vi "RTM Frames to be Faulted.vi"(8 "error in (no error)":errorcluster) -> (0 "error out":errorcluster)   [LabVIEW 2018, in "CAN Gateway System Explorer.lvlib"]
uses:
  CAN Gateway System Explorer.lvlib
  <vilib>/NI Veristand/Custom Device API/Custom Device Item Ref.ctl
  <vilib>/NI Veristand/Custom Device API/Custom Device API.lvlib
panel:
  out "Node Ptr 2":T1 format="%.0x"
  in  "Node Ptr":T1 format="%.0x"
  in  "Tag":string
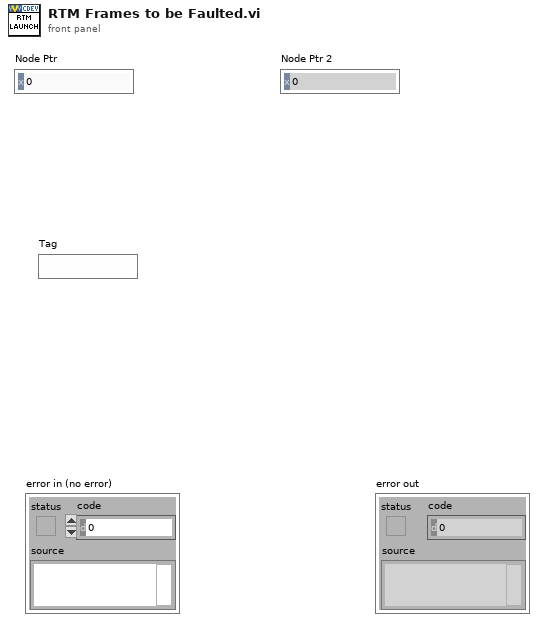
[diagram p1: front panel]
types:
  T1 = typedef "Custom Device API.lvlib/Custom Device Item Ref.ctl" = u64
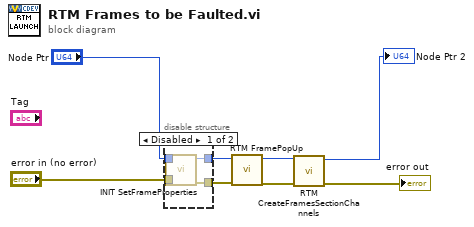
[diagram p0: block diagram]
diagram:
  n1 = disable-structure shown="Disabled" {
    disable-tunnel: [w12 w13] -> w5
    disable-tunnel: "error in (no error)" -> [w11 w13]
    disable-tunnel: "Node Ptr" -> [w10 w14]
    disable-tunnel: [w9 w14] -> w2
    frame Disabled {
      n2 = call "INIT SetFrameProperties.vi"("error in (no error)"=w11, "Device Item Ref in"=w10) -> ("error out"=w12:errorcluster, "Device Item Ref out"=w9:T1)  [unwired: 8 in]
    }
    frame Enabled {
    }
  }
  n3 = call "RTM FramePopUp.vi"("error in (no error)"=w5, "Node Ptr"=w2) -> ("error out"=w8:errorcluster, "Node Ptr 2"=w1:T1)  [unwired: 8 in]
  n4 = call "RTM CreateFramesSectionChannels.vi"("error in (no error)"=w8, "Node Ptr"=w1) -> ("error out"=→"error out":errorcluster, "Node Ptr 2"=→"Node Ptr 2":T1)  [unwired: 8 in]
